vi "Untitled 2.vi"(8 "error in (no error)":errorcluster, 11 "Collection in":refnum<class "Collection.lvclass">=refnum) -> (0 "error out":errorcluster, 2 "Area":T1, 3 "Collection out":refnum<class "Collection.lvclass">)   [LabVIEW 2020]
uses:
  Collection/Collection.lvclass
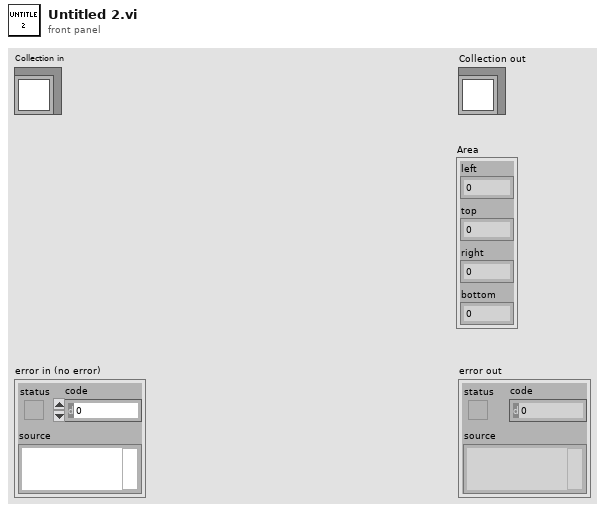
[diagram p1: front panel]
types:
  T1 = cluster{"left":i16, "top":i16, "right":i16, "bottom":i16}
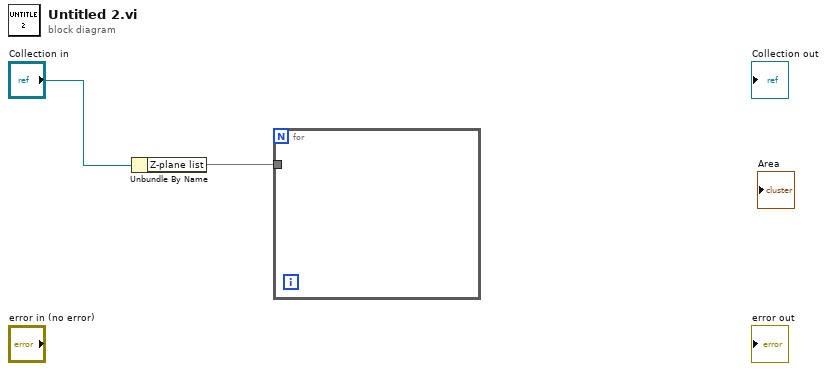
[diagram p0: block diagram]
diagram:
  n1 = Unbundle By Name("Collection in") -> ("Z-plane list"=w1)
  n2 = for {
    tunnel: w1 -> [_]
  }
